vi "Connect.vi"(8 "error in":errorcluster, 11 "Axis in":refnum<class "Axis.lvclass">) -> (0 "error out":errorcluster, 3 "Axis out":refnum<class "Axis.lvclass">)   [LabVIEW 2018, in "Axis.lvlib" / "Axis.lvclass"]
uses:
  Axis.lvclass
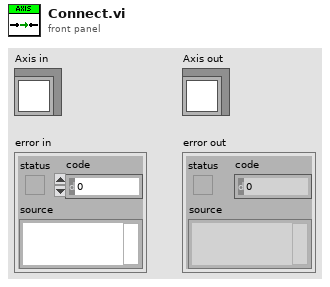
[diagram p1: front panel]
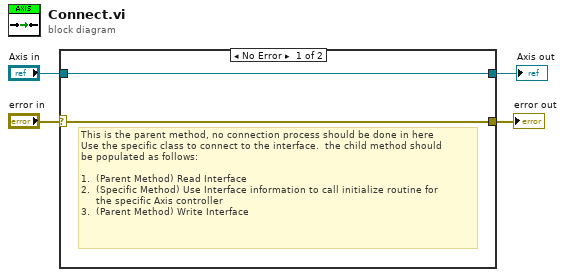
[diagram p0: block diagram]
diagram:
  n1 = case shown="No Error" "error in" {
    selector: "error in" -> [w5 w8]
    tunnel: [w5 w8] -> w3
    tunnel: [w6 w7] -> w1
    tunnel: "Axis in" -> [w6 w7]
    frame No Error {
      # "This is the parent method, no connection process should be done in here\nUse the specific class to connect to the interface.  the child method should \nbe populated as follows:\n\n1.  (Parent Method) Read Interface\n2.  (Specific Method) Use Interface information to call initialize routine for \n     the specific Axis controller \n3.  (Parent Method) Write Interface"
    }
    frame Error {
    }
  }
  "error out" <- w3
  "Axis out" <- w1
